vi "Delete_Internal_TargetFileDir_On_Error.vi"(8 "error in (no error)":errorcluster, 10 "override Mac support directory preservation":bool, 11 "Build in":refnum<class "AB_Targetfile.lvclass">) -> (0 "error out":errorcluster, 3 "Build out":refnum<class "AB_Targetfile.lvclass">)   [LabVIEW 2020, in "AB_Targetfile.lvclass"]
uses:
  <vilib>/AppBuilder/AB_Classes/TargetFile/AB_Targetfile.lvclass
  e:/builds/penguin/labview/branches/2020/dev/dist/vi.lib/AppBuilder/AB_Classes/Build/AB_Build.lvclass
  <vilib>/AppBuilder/AB_Classes/TargetFile/AB_Targetfile.lvclass/AB_Targetfile.ctl
  <vilib>/AppBuilder/AB_Classes/Build/AB_Build.lvclass
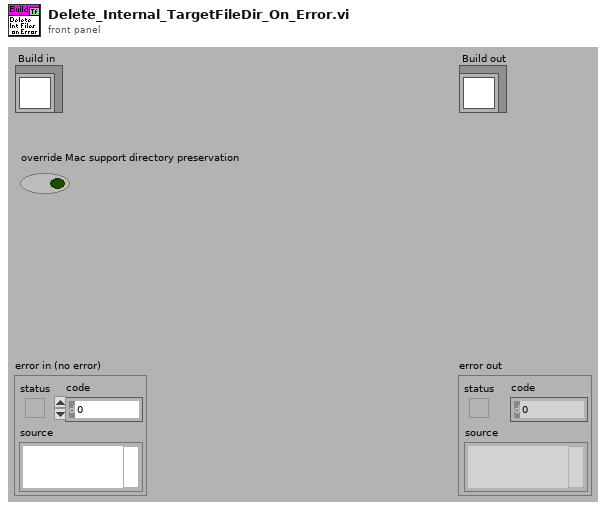
[diagram p1: front panel]
types:
  T1 = typedef "AB_Build.ctl" = cluster{"buildSpecName":string, "buildSpecDescription":string, "destinations":refnum<class "AB_Destination.lvclass">[], "exclusionOption":T2, "defaultLanguage":string, "supportedLanguages":string[], "excludedDirectories":path[], "buildContext":refnum<vi>, "buildObject":T3, "preview":bool, "programatic":bool, "progressBarEvents":T4, "userLog_Path":path, "preActionID":string, "preAction_Path":path, "postActionID":string, "postAction_Path":path, "eng_checkForBrokenVIs?":bool, "eng_verboseLinkerErrors?":bool, "localDest_Path":path, "targetDest_Path":path, "removeVIObject":u16, "cache":refnum<class "PreviewCache.lvclass">, "use cache":bool, "previewCache_ID":string, "buildCache_ID":string, "eng_TempLocalDest_Path":path, "eng_collectDependencies?":bool, "versionInfo":cluster{"buildVersion":cluster{"major":u16, "minor":u16, "patch":u16, "build":u16}, "autoIncrement":bool}, "eng_enableVIChecksums":bool}
  T2 = typedef "AB_Exclusion_Option.ctl" = cluster{"typedefs":bool, "polymorphicVIs":bool, "unusedLibraryItems":bool, "modifyLibraryFile":bool, "edit-timeDependencies":bool, "inlineVIs":bool, "dependent PPLs":bool, "dependent DLLs":bool}
  T3 = typedef "ItemRef.ctl" = u64
  T4 = typedef "provcom_ProgressBar_Events.ctl" = cluster{"newJob":refnum<user-event>, "newItem":refnum<user-event>, "errorMsg":T5, "cancel":refnum<user-event>}
  T5 = typedef "mxLvBuildError.ctl" = refnum<user-event>
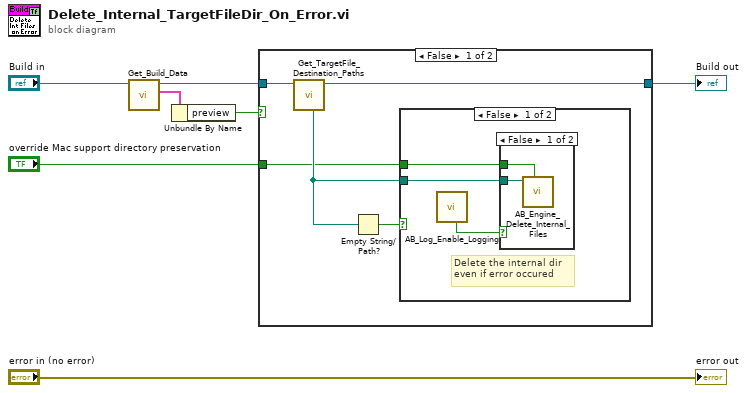
[diagram p0: block diagram]
diagram:
  n1 = call <vilib>:"Get_Build_Data.vi"("Class in"="Build in") -> ("data"=w3:T1, "Class out"=w4:refnum<class "AB_Targetfile.lvclass">)  [unwired: 8 in, 1 out]
  n2 = Unbundle By Name(w3) -> ("preview"=w2:bool)
  n3 = case shown="False" w2 {
    tunnel: [w12 w18] -> w6
    tunnel: w4 -> [w11 w18]
    tunnel: "override Mac support directory preservation" -> [w8 _]
    frame False {
      n4 = call <vilib>:"Get_TargetFile_Destination_Paths.vi"("AB_Targetfile in"=w11) -> ("AB_Targetfile out"=w12:refnum<class "AB_Targetfile.lvclass">, "targetfile path"=w10:path)  [unwired: 1 in, 8 out]
      n5 = Empty String/Path?(string/path=w10) -> (empty?=w9:bool)
      n6 = case shown="False" w9 {
        tunnel: w10 -> [w14 _]
        tunnel: w8 -> [w13 _]
        frame False {
          # "Delete the internal dir even if error occured"
          n7 = call <vilib>:"AB_Log_Enable_Logging.vi"() -> ("keep internal.llb"=w15:bool)  [unwired: 2 in, 9 out]
          n8 = case shown="False" w15 {
            tunnel: w14 -> [w17 _]
            tunnel: w13 -> [w16 _]
            frame False {
              n9 = call <vilib>:"AB_Engine_Delete_Internal_Files.vi"("override Mac support directory preservation"=w16, "internal directory"=w17) -> ()  [unwired: 2 in, 8 out]
            }
            frame True {
            }
          }
        }
        frame True {
        }
      }
    }
    frame True {
      # "Don't do anything if this is a preview."
    }
  }
  "Build out" <- w6
  "error out" <- "error in (no error)"
